vi "Untitled 1.vi"() -> ()   [LabVIEW 2022 SP3]
panel:
  out "resulting string":string
  in  "Temprature":dbl
  in  "B":i8
  in  "A":i8
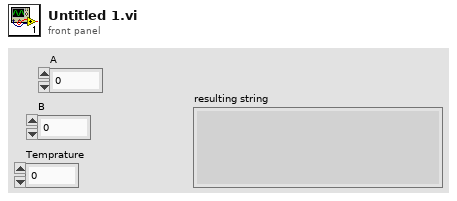
[diagram p1: front panel]
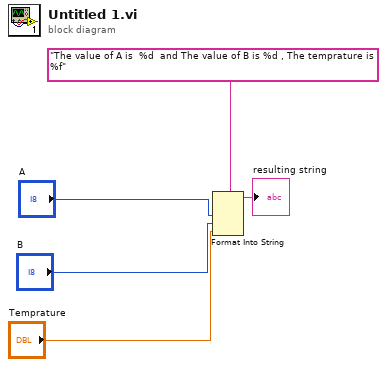
[diagram p0: block diagram]
diagram:
  n1 = Format Into String(format string="The value of A is  %d  and The value of B is %d , The temprature is %f", "A", "B", "Temprature") -> (resulting string=→"resulting string":string)  [unwired: 2 in, 1 out]
